vi "XSP3_GetFrame.vi"(8 "ErrorIn":errorcluster, 11 "ProcessIn":string="XSPRESS3-EXAMPLE" caption="ProcessName") -> (0 "ErrorOut":errorcluster, 2 "Status":bool, 3 "ProcessOut":string caption="ProcessName", 4 "Frame":i32 caption="FrameReadout")   [LabVIEW 2010]
uses:
  Program Files/National Instruments/LabVIEW 2017/user.lib/caLab/Private/Get_PV.vi
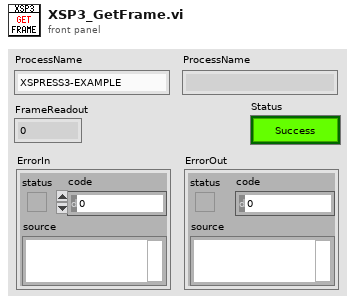
[diagram p1: front panel]
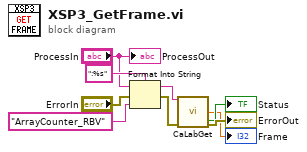
[diagram p0: block diagram]
diagram:
  n1 = Format Into String(format string=":%s" ("PV"), initial string="ProcessIn", error in="ErrorIn", "ArrayCounter_RBV" ("PV")) -> (resulting string=w2:string, error out=w3:errorcluster)
  n2 = call-poly "CaLabGet.vi"("PV Name"=w2, "Error in (no error)"=w3) -> ("1rst Value (number)"=→"Frame":dbl, "Status"=→"Status":bool, "Error out"=→"ErrorOut":errorcluster)  [unwired: 7 in, 4 out]
  "ProcessOut" <- "ProcessIn"
